vi "Logger.File.Read.vi"(8 "error in (no error)":errorcluster, 9 "Update Stats (F)":bool, 11 "file path":path) -> (0 "error out":errorcluster, 1 "Stats elements":i32, 2 "File content":T1, 3 "Ref":string)   [LabVIEW 2016]
uses:
  Logger.File.ctl
  Logger.File.Properties.ctl
  Sequence/Sequence.Code.SerialFormat.ctl
  Sequence/Sequence.Counters.ctl
  Logger.File.Serials.ctl
  Sequence/Sequence.Step.Status.ctl
  Logger.Stats.Fglb.Action.ctl
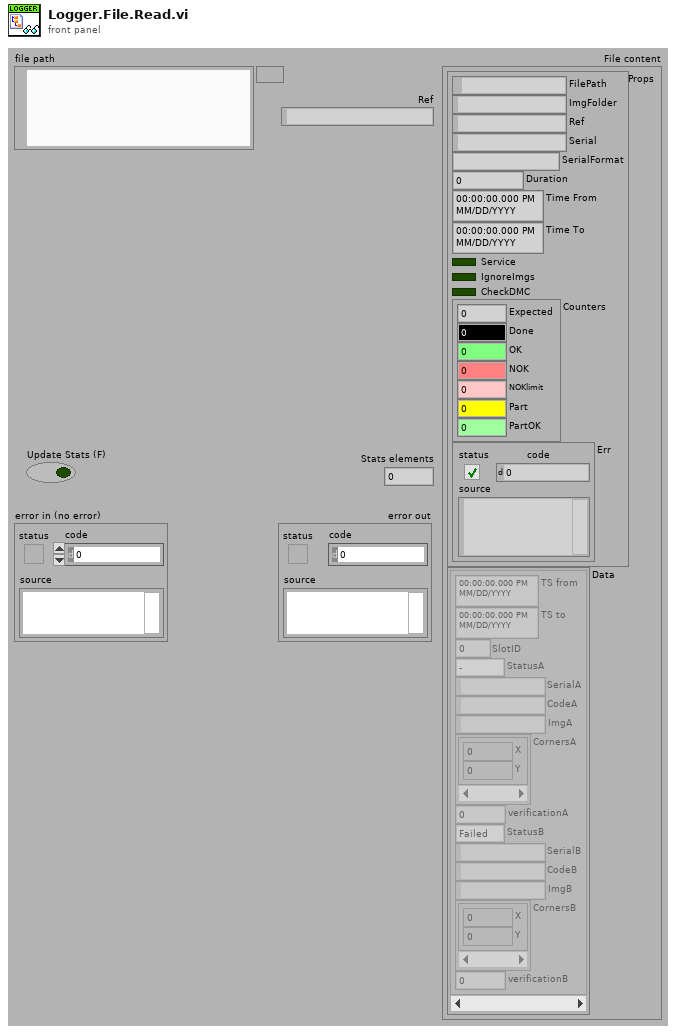
[diagram p1: front panel]
types:
  T1 = typedef "Logger.File.ctl" = cluster{"Props":T2, "Data":T5[]}
  T2 = typedef "Logger.File.Properties.ctl" = cluster{"FilePath":path, "ImgFolder":string, "Ref":string, "Serial":string, "SerialFormat":T3, "Duration":dbl, "Time From":timestamp, "Time To":timestamp, "Service":bool, "IgnoreImgs":bool, "CheckDMC":bool, "Counters":T4, "Err":errorcluster}
  T3 = typedef "Sequence.Code.SerialFormat.ctl" = enum8{"", "6 dig", "7 dig"}
  T4 = typedef "Sequence.Counters.ctl" = cluster{"Expected":u16, "Done":u16, "OK":u16, "NOK":u16, "NOKlimit":u16, "Part":u16, "PartOK":u16}
  T5 = typedef "Logger.File.Serials.ctl" = cluster{"TS from":timestamp, "TS to":timestamp, "SlotID":u8, "StatusA":T6, "SerialA":string, "CodeA":string, "ImgA":string, "CornersA":cluster{"X":i32, "Y":i32}[], "verificationA":u8, "StatusB":T6, "SerialB":string, "CodeB":string, "ImgB":string, "CornersB":cluster{"X":i32, "Y":i32}[], "verificationB":u8}
  T6 = typedef "Sequence.Step.Status.ctl" = enum16{"-", "Pending", "Running", "Skipped", "Passed", "Failed", "Done", "Error", "Aborted", "Stopped"}
  T7 = typedef "Logger.Stats.Fglb.Action.ctl" = enum16{"init", "add", "get", "get all"}
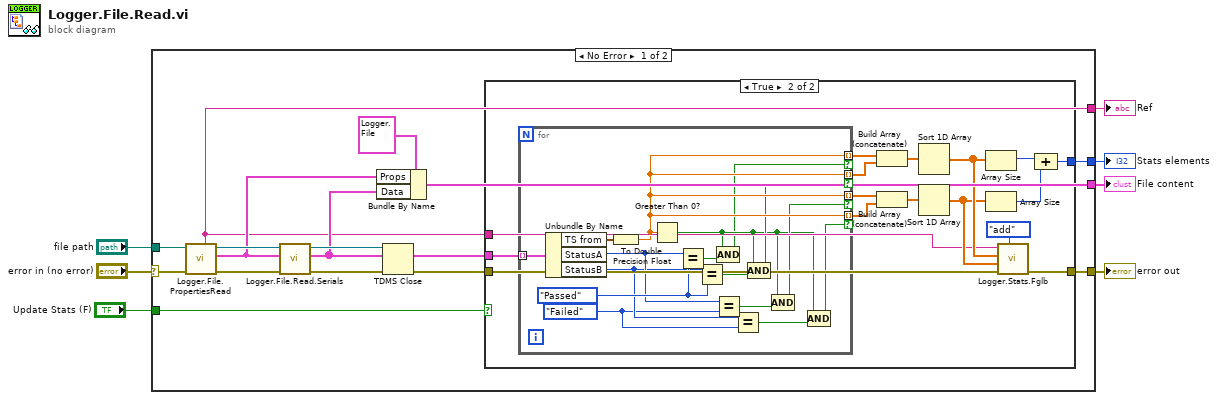
[diagram p0: block diagram]
diagram:
  n1 = case shown="No Error" "error in (no error)" {
    selector: "error in (no error)" -> [w21 w56]
    tunnel: [w10 w56] -> w5
    tunnel: "file path" -> [w22 _]
    tunnel: [w17 _] -> w4
    tunnel: [w11 _] -> w3
    tunnel: "Update Stats (F)" -> [w9 _]
    tunnel: [w8 _] -> w1
    frame No Error {
      n2 = call "Logger.File.PropertiesRead.vi"("error in (no error)"=w21, "file path"=w22) -> ("error out"=w20:errorcluster, "Properties"=w14:T2, "File ref out"=w19:refnum<k34>, "Ref"=w11:string)  [unwired: 6 in]
      n3 = call "Logger.File.Read.Serials.vi"("error in"=w20, "Properties"=w14, "file ref in"=w19) -> ("error out"=w15:errorcluster, "Data"=w12:T5[], "file ref out"=w16:refnum<k34>)  [unwired: 6 in]
      n4 = Bundle By Name(cluster=T1 {"Props"={"FilePath"=path "", "ImgFolder"="", "Ref"="", "Serial"="", "SerialFormat"=enum."", "Duration"=0.0, "Time From"=timestamp(0 s since 1904-01-01), "Time To"=timestamp(0 s since 1904-01-01), "Service"=FALSE, "IgnoreImgs"=FALSE, "CheckDMC"=FALSE, "Counters"={"Expected"=0, "Done"=0, "OK"=0, "NOK"=0, "NOKlimit"=0, "Part"=0, "PartOK"=0}, "Err"={"status"=FALSE, "code"=0, "source"=""}}, "Data"=[]} ("Properties"), "Props"=w14, "Data"=w12) -> (w17:T1)
      n5 = TDMS Close(8:w15, 11:w16) -> (0:w13:errorcluster)  [unwired: 1 out]
      n6 = case shown="True" w9 {
        tunnel: w13 -> [w23 w28]
        tunnel: w12 -> [_ w27]
        tunnel: w11 -> [_ w24]
        tunnel: [w23 w26] -> w10
        tunnel: [_ w25] -> w8
        frame False {
        }
        frame True {
          n7 = for {
            tunnel: w27 -> [w55] mode=indexing
            tunnel: [w49] -> w39 mode=indexing if=w40
            tunnel: [w49] -> w37 mode=indexing if=w43
            tunnel: [w49] -> w35 mode=indexing if=w45
            tunnel: [w49] -> w34 mode=indexing if=w47
            w51 = Sequence.Step.Status."Failed" ("y")
            w54 = Sequence.Step.Status."Passed" ("y")
            n8 = Unbundle By Name(w55) -> ("TS from"=w50:timestamp, "StatusA"=w53:T6, "StatusB"=w52:T6)
            n9 = To Double Precision Float(number=w50) -> (double precision float=w49:dbl)
            n10 = Greater Than 0?(x=w49) -> (x > 0?=w41:bool)
            n11 = Equal?(x=w53, y=w54) -> (x = y?=w42:bool)
            n12 = Equal?(x=w52, y=w54) -> (x = y?=w44:bool)
            n13 = Equal?(x=w53, y=w51) -> (x = y?=w46:bool)
            n14 = Compound Arithmetic op=AND(w41, w42) -> (w40:bool)
            n15 = Equal?(x=w52, y=w51) -> (x = y?=w48:bool)
            n16 = Compound Arithmetic op=AND(w41, w44) -> (w43:bool)
            n17 = Compound Arithmetic op=AND(w41, w46) -> (w45:bool)
            n18 = Compound Arithmetic op=AND(w41, w48) -> (w47:bool)
          }
          n19 = Build Array (concatenate)(w39, w37) -> (w38:dbl[])
          n20 = Build Array (concatenate)(w35, w34) -> (w36:dbl[])
          n21 = Sort 1D Array(array=w38) -> (sorted array=w32:dbl[])
          n22 = Sort 1D Array(array=w36) -> (sorted array=w31:dbl[])
          n23 = Array Size(array=w32) -> (size(s)=w30:i32)
          n24 = Array Size(array=w31) -> (size(s)=w29:i32)
          n25 = call "Logger.Stats.Fglb.vi"("Action (get)"=Logger.Stats.Fglb.Action."add" ("Action"), "error in (no error)"=w28, "dbg_NOK"=w31, "dbg_OK"=w32, "Variant"=w24) -> ("error out"=w26:errorcluster)  [unwired: 5 in, 1 out]
          n26 = Compound Arithmetic op=ADD(w30, w29) -> (w25:i32)
        }
      }
    }
    frame Error {
    }
  }
  "error out" <- w5
  "File content" <- w4
  "Ref" <- w3
  "Stats elements" <- w1
